vi "FITS_Find_Keyword.vi"(0 "FITS bytes":string, 1 "Keyword":string) -> (2 "raw string":string, 3 "I32 value":i32, 4 "DBL value":dbl, 5 "Found ?":bool=TRUE)   [LabVIEW 2020]
panel:
  out "after substring":string
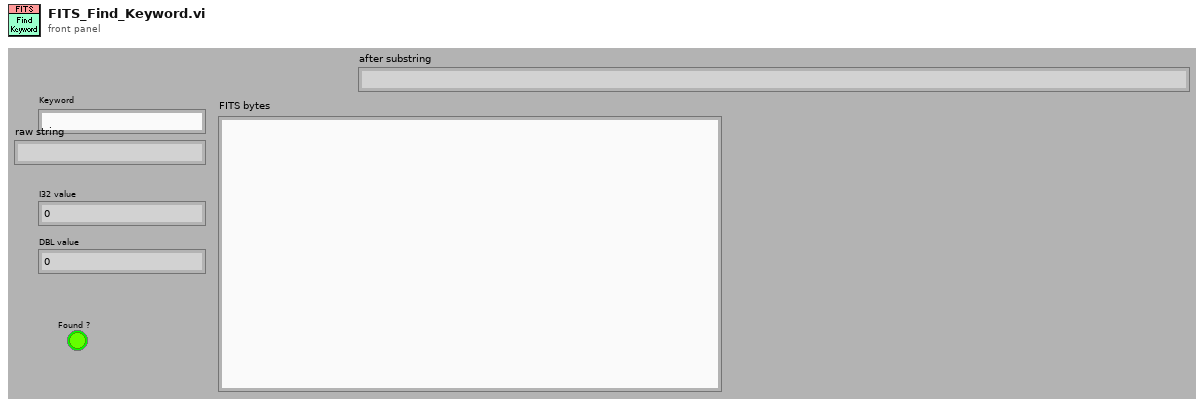
[diagram p1: front panel]
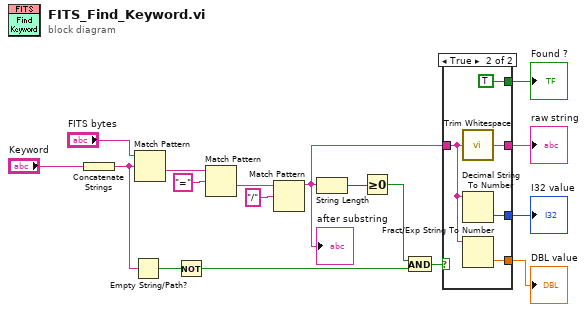
[diagram p0: block diagram]
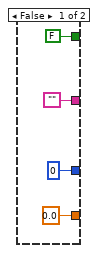
[diagram p2: hidden frame]
diagram:
  n1 = Concatenate Strings("Keyword") -> (w7:string)
  n2 = Empty String/Path?(string/path=w7) -> (empty?=w15:bool)
  n3 = Match Pattern(string="FITS bytes", regular expression=w7) -> (after substring=w6:string)  [unwired: 1 in, 3 out]
  n4 = Not(x=w15) -> (.not. x?=w13:bool)
  n5 = Match Pattern(string=w6, regular expression="=") -> (after substring=w4:string)  [unwired: 1 in, 3 out]
  n6 = Match Pattern(string=w4, regular expression="/") -> (before substring=w2:string)  [unwired: 1 in, 3 out]
  "after substring" <- w2
  n7 = String Length(string=w2) -> (length=w1:i32)
  n8 = Greater Or Equal To 0?(x=w1) -> (x >= 0?=w14:bool)
  n9 = And(x=w14, y=w13) -> (x .and. y?=w12:bool)
  n10 = case shown="True" w12 {
    tunnel: w2 -> [_ w22]
    tunnel: [FALSE TRUE] -> w16
    tunnel: ["" w25] -> w11
    tunnel: [0 w24] -> w10
    tunnel: [0.0 w23] -> w9
    frame False {
    }
    frame True {
      n11 = call <vilib>:"Trim Whitespace.vi"("string"=w22) -> ("trimmed string"=w25:string)  [unwired: 1 in]
      n12 = Decimal String To Number(string=w22) -> (number=w24:i32)  [unwired: 2 in, 1 out]
      n13 = Fract/Exp String To Number(string=w22) -> (number=w23:dbl)  [unwired: 3 in, 1 out]
    }
  }
  "Found ?" <- w16
  "I32 value" <- w10
  "raw string" <- w11
  "DBL value" <- w9
